vi "draw.vi"(0 "reference":refnum<class "StateDiagramGraph.lvclass">, 1 "graphics":refnum<class "Graphics.lvclass">, 2 "grid":refnum<class "Grid.lvclass">, 5 "error in (no error)":errorcluster, 6 "SelectedNodes":refnum<class "AbstractNode.lvclass">[](array[class]), 7 "HideOverLays(False)":bool) -> (14 "reference out":refnum<class "StateDiagramGraph.lvclass">, 15 "NodesBounds":T4 {"height" format="%.2f"; "width" format="%.2f"; "y" format="%.2f"; "x" format="%.2f"}, 16 "HotSpots":T1[](array[typedef]) {"HotSpot"."y" format="%.2f"; "HotSpot"."x" format="%.2f"}, 19 "error out":errorcluster)   [LabVIEW 2020, in "StateDiagramGraph.lvclass"]
doc: "draw"
uses:
  <resource>/Framework/Providers/Open_GDS/UML/StateDiagramGraph_class/StateDiagramGraph.lvclass
  <resource>/Framework/Providers/Open_GDS/UML/Graphics_class/Graphics.lvclass
  <resource>/Framework/Providers/Open_GDS/UML/Grid_class/Grid.lvclass
  <resource>/Framework/Providers/Open_GDS/UML/General/Rectangle/Rectangle Rectangle2D.ctl
  <resource>/Framework/Providers/Open_GDS/UML/AbstractNode_class/AbstractNode.lvclass
  <resource>/Framework/Providers/Open_GDS/UML/UMLEditor/UMLEditor_HotSpotData.ctl
  <resource>/Framework/Providers/Open_GDS/UML/General/Point/Point Point2D.ctl
  <resource>/Framework/Providers/Open_GDS/UML/UMLEditor/UMLEditor_HotSpotType.ctl
  <resource>/Framework/Providers/Open_GDS/UML/StateDiagramGraph_class/private/ViPathShowOption.ctl
  <resource>/Framework/Providers/Open_GDS/UML/Graphics_class/FontType.ctl
  <resource>/Framework/Providers/Open_GDS/UML/Graph_class/Graph.lvclass
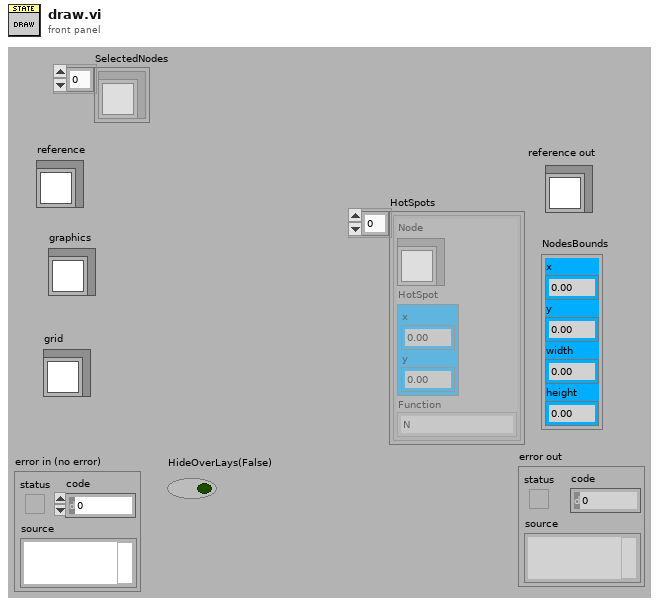
[diagram p1: front panel]
types:
  T1 = typedef "UMLEditor_HotSpotData.ctl" = cluster{"Node":refnum<class "AbstractNode.lvclass">, "HotSpot":T2, "Function":T3}
  T2 = typedef "Point Point2D.ctl" = cluster{"x":dbl, "y":dbl}
  T3 = typedef "UMLEditor_HotSpotType.ctl" = enum16{"N", "NE", "E", "SE", "S", "SW", "W", "NW", "Expand", "Collaps"}
  T4 = typedef "Rectangle Rectangle2D.ctl" = cluster{"x":dbl, "y":dbl, "width":dbl, "height":dbl}
  T5 = typedef "StateDiagramGraph.lvclass/ViPathShowOption.ctl" = enum16{"Don't Show", "Show Relative Path", "Show Absolute Path"}
  T6 = typedef "Graphics.lvclass/FontType.ctl" = cluster{"Font Name:":string, "Size":i16, "Strikeout?":bool, "Italic?":bool, "Underline?":bool, "Outline?":bool, "Shadow?":bool, "Bold?":bool}
  T7 = typedef "StateDiagramGraph.lvclass/ObjectAttributes.ctl" = cluster{"StateDiagramData":T8}
  T8 = typedef "StateDiagramGraph.lvclass/StateDiagramData.ctl" = cluster{"VI-Path":path, "ShowOption":T5}
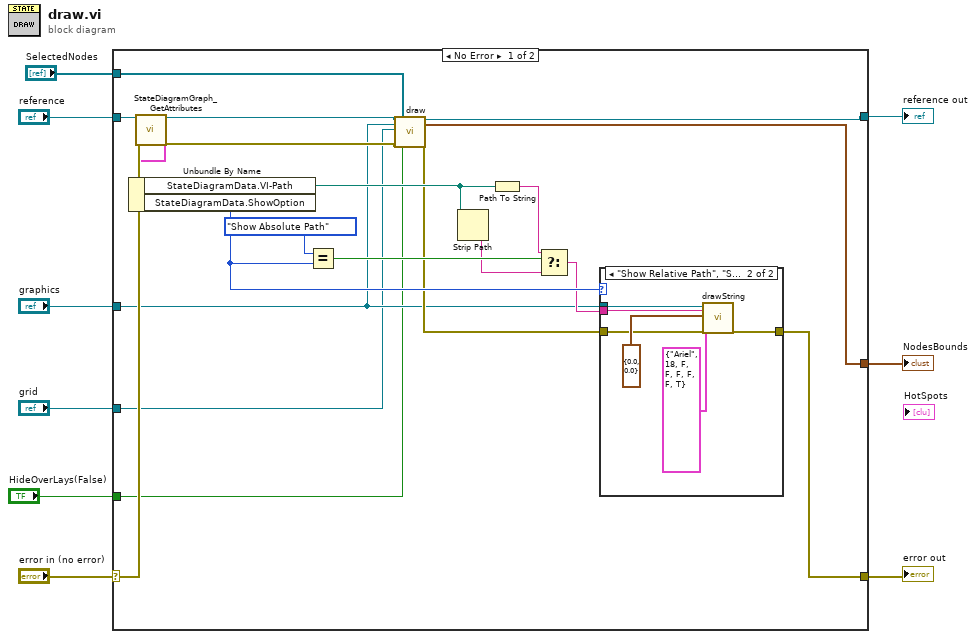
[diagram p0: block diagram]
diagram:
  n1 = case shown="No Error" "error in (no error)" {
    selector: "error in (no error)" -> [w29 w37]
    tunnel: "reference" -> [w28 w38]
    tunnel: [w27 w37] -> w7
    tunnel: [w16 w38] -> w6
    tunnel: "graphics" -> [w15 _]
    tunnel: "grid" -> [w14 _]
    tunnel: [w13 _] -> w3
    tunnel: "SelectedNodes" -> [w12 _]
    tunnel: "HideOverLays(False)" -> [w11 _]
    frame No Error {
      n2 = call <resource>:"StateDiagramGraph_GetAttributes.vi"("reference in"=w28, "error in (no error)"=w29) -> ("reference out"=w19:refnum<class "StateDiagramGraph.lvclass">, "Data"=w10:T7, "error out"=w18:errorcluster)  [unwired: 1 in, 14 out]
      n3 = Unbundle By Name(w10) -> ("StateDiagramData.VI-Path"=w21:path, "StateDiagramData.ShowOption"=w26:T5)
      n4 = Equal?(x=ViPathShowOption."Show Absolute Path", y=w26) -> (x = y?=w24:bool)
      n5 = call-parent "draw.vi"("reference"=w19, "graphics"=w15, "grid"=w14, "error in (no error)"=w18, "SelectedNodes"=w12, "HideOverLays(False)"=w11) -> ("reference out"=w16:refnum<class "StateDiagramGraph.lvclass">, "NodesBounds"=w13:T4, "error out"=w17:errorcluster)  [unwired: 10 in, 1 out]
      n6 = Strip Path(path=w21) -> (name=w20:string)  [unwired: 1 out]
      n7 = Path To String(path=w21) -> (string=w23:string)
      n8 = Select(t=w23, s=w24, f=w20) -> (s? t:f=w22:string)
      n9 = case shown="\"Show Relative Path\", \"Show Absolute Path\"" w26 {
        tunnel: w15 -> [_ w36]
        tunnel: w22 -> [_ w35]
        tunnel: [w30 w34] -> w27
        tunnel: w17 -> [w30 w31]
        frame "Don't Show", Default {
        }
        frame "Show Relative Path", "Show Absolute Path" {
          n10 = call-dynamic "drawString.vi"("reference"=w36, "text"=w35, "textPos"=T2 {"x"=0.0, "y"=0.0}, "font"=T6 {"Font Name:"="Ariel", "Size"=18, "Strikeout?"=FALSE, "Italic?"=FALSE, "Underline?"=FALSE, "Outline?"=FALSE, "Shadow?"=FALSE, "Bold?"=TRUE}, "error in (no error)"=w31) -> ("error out"=w34:errorcluster)  [unwired: 13 in, 1 out]
        }
      }
    }
    frame Error {
    }
  }
  "reference out" <- w6
  "error out" <- w7
  "NodesBounds" <- w3
